vi "Load Column Headers.vi"(8 "error in (no error)":errorcluster, 11 "Standard Display Configuration in":refnum<class "Standard Display Configuration.lvclass">) -> (0 "error out":errorcluster, 3 "Standard Display Configuration out":refnum<class "Standard Display Configuration.lvclass">)   [LabVIEW 2016, in "Assert API Components.lvlib" / "Assert Display.lvlib" / "Main Display.lvlib" / "Standard Display Configuration.lvclass"]
uses:
  Standard Display Configuration.lvclass
  D:/Work/Projects/actor_assert_api/Core/Main Display/Display Configurations/Base Display Configuration.lvclass
  Base Display Configuration.lvclass/Base Display Configuration.ctl
  <vilib>/Utility/config.llb/Read Key (String).vi
  Assert API Components/Assert API Components.lvlib
  <vilib>/Utility/config.llb/NI_LVConfig.lvlib
  Base Display Configuration.lvclass
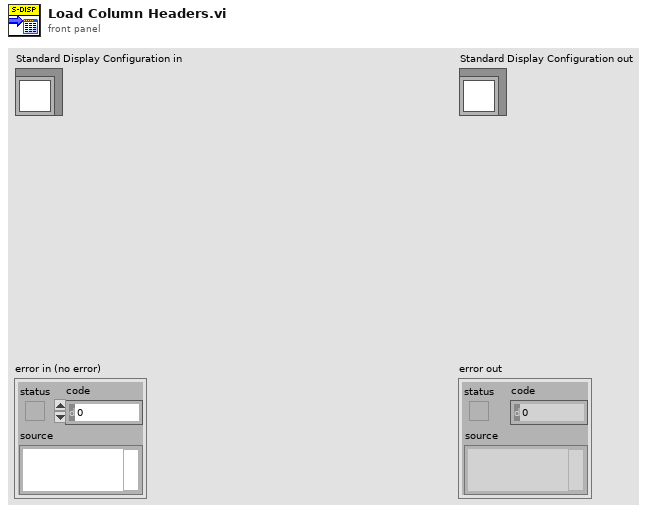
[diagram p1: front panel]
types:
  T1 = typedef "NI_LVConfig.lvlib/Config Data RefNum.ctl" = refnum<k1>
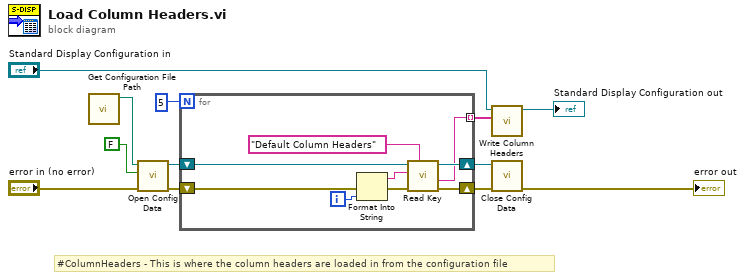
[diagram p0: block diagram]
diagram:
  # "#ColumnHeaders - This is where the column headers are loaded in from the configuration file"
  n1 = call "Get Configuration File Path.vi"() -> ("Configuration File Path"=w5:path)  [unwired: 11 in]
  n2 = call <vilib>:"Open Config Data.vi"("error in (no error)"="error in (no error)", "create file if necessary (T)"=FALSE, "configuration file path"=w5) -> ("error out"=w10:errorcluster, "refnum"=w7:T1)  [unwired: 6 in, 1 out]
  n3 = for {
    N: 5 -> [_]
    shift-right: [w21] -> w9
    shift-left: w10 -> [w14]
    shift-right: [w19] -> w6
    shift-left: w7 -> [w20]
    tunnel: [w15] -> w1 mode=indexing
    i -> [w17]
    n4 = Format Into String(error in=w14, w17) -> (resulting string=w16:string, error out=w13:errorcluster)  [unwired: 2 in]
    n5 = call-poly <vilib>:"Read Key.vi"("section"="Default Column Headers", "error in (no error)"=w13, "key"=w16, "refnum"=w20) -> ("error out"=w21:errorcluster, "value"=w15:string, "refnum out"=w19:T1)  [unwired: 4 in, 1 out]
  }
  n6 = call "Write Column Headers.vi"("Column Headers"=w1, "Base Display Configuration in"="Standard Display Configuration in") -> ("Base Display Configuration out"=→"Standard Display Configuration out":refnum<class "Standard Display Configuration.lvclass">)  [unwired: 9 in]
  n7 = call <vilib>:"Close Config Data.vi"("error in (no error)"=w9, "refnum"=w6) -> ("error out"=→"error out":errorcluster)  [unwired: 8 in, 1 out]
